vi "oa_Check Time or RPM Segment.vi"(11 "range in":cluster{"start":dbl, "end":dbl, "step":dbl} {"step" format="%.2f"; "end" format="%.2f"; "start" format="%.2f"}) -> (1 "empty?":bool, 3 "range out":cluster{"start":dbl, "end":dbl, "step":dbl} {"step" format="%.2f"; "end" format="%.2f"; "start" format="%.2f"})   [LabVIEW 2017, in "SoundVib_Resampling.lvlib"]
uses:
  <vilib>/addons/Sound and Vibration/Order Analysis/Resample Order Tracking/SoundVib_Resampling.lvlib
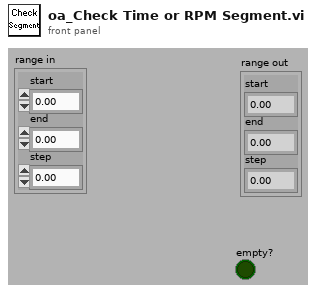
[diagram p1: front panel]
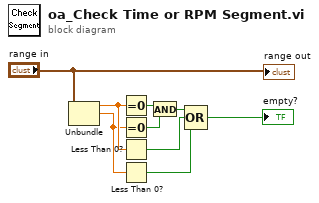
[diagram p0: block diagram]
diagram:
  n1 = Unbundle("range in") -> ("start"=w6:dbl, "end"=w5:dbl)  [unwired: 1 out]
  n2 = Equal To 0?(x=w6) -> (x = 0?=w8:bool)
  n3 = Equal To 0?(x=w5) -> (x = 0?=w7:bool)
  n4 = Less Than 0?(x=w6) -> (x < 0?=w3:bool)
  n5 = Less Than 0?(x=w5) -> (x < 0?=w2:bool)
  n6 = And(x=w8, y=w7) -> (x .and. y?=w4:bool)
  n7 = Compound Arithmetic op=OR(w4, w3, w2) -> (→"empty?":bool)
  "range out" <- "range in"
